vi "LV SciSDK INIT OSCILLOSCOPE.vi"(0 "Oscilloscope Name":string, 1 "Trigger Mode":string(combo)="self", 2 "Decimator":u32, 3 "Timeout":dbl=5000.0, 4 "Handle In":T2, 5 "error in (no error)":errorcluster, 6 "Pretrigger":u32, 7 "Acq Mode":string(combo)="blocking", 8 "Trigger Level":u32, 9 "Trigger Channel":u32, 10 "Trigger Polarity":string(combo)="pos", 11 "Auto Arm":u32=1) -> (18 "Oscilloscope Handle Out":T1, 19 "error out":errorcluster)   [LabVIEW 2021]
uses:
  SciSDK_Labview.lvlib
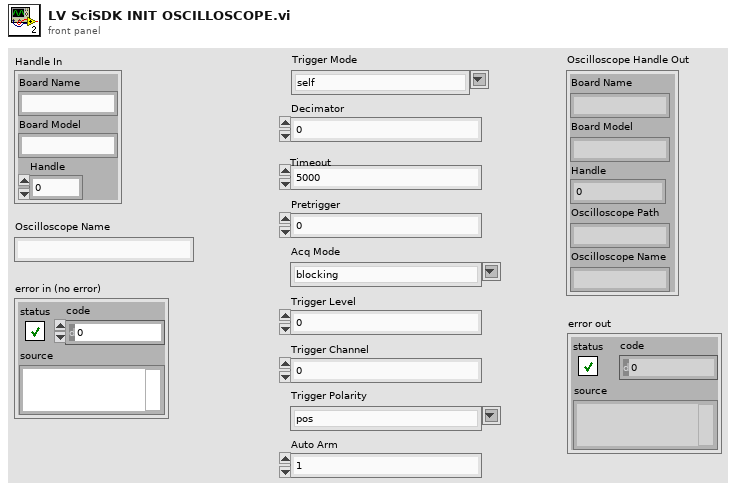
[diagram p1: front panel]
types:
  T1 = cluster{"Board Name":string, "Board Model":string, "Handle":u64, "Oscilloscope Path":string, "Oscilloscope Name":string}
  T2 = cluster{"Board Name":string, "Board Model":string, "Handle":u64}
  T3 = cluster{"Board Name":string, "Board Model":string, "Handle":u64, string, "Oscilloscope Name":string}
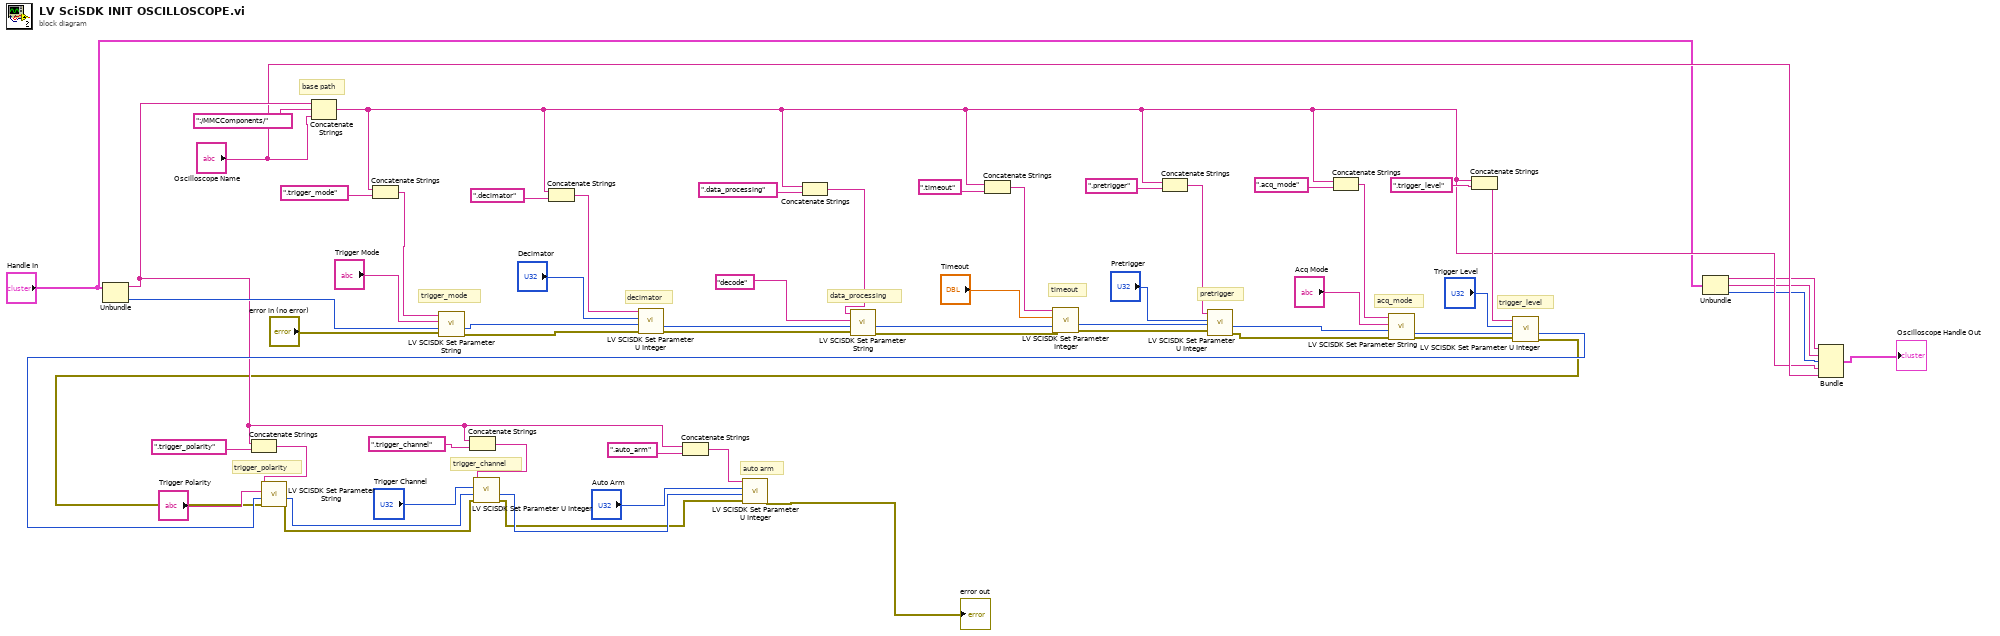
[diagram p0: block diagram]
diagram:
  # "auto arm"
  # "trigger_polarity"
  # "trigger_channel"
  # "trigger_level"
  # "acq_mode"
  # "pretrigger"
  # "base path"
  # "timeout"
  # "data_processing"
  # "decimator"
  # "trigger_mode"
  n1 = Unbundle("Handle In") -> ("Board Name"=w21:string, "Handle"=w60:u64)  [unwired: 1 out]
  n2 = Concatenate Strings(w21, ".trigger_polarity" ("string")) -> (w34:string)
  n3 = Concatenate Strings(w21, ":/MMCComponents/" ("string"), "Oscilloscope Name") -> (w17:string)
  n4 = Concatenate Strings(w17, ".trigger_mode" ("string")) -> (w54:string)
  n5 = call "LV SCISDK Set Parameter String.vi"("error in (no error)"="error in (no error)", "handle"=w60, "value"="Trigger Mode", "Path"=w54) -> ("error out"=w10:errorcluster, "handle out"=w59:u64)  [unwired: 5 in, 1 out]
  n6 = Concatenate Strings(w21, ".trigger_channel" ("string")) -> (w36:string)
  n7 = Concatenate Strings(w17, ".decimator" ("string")) -> (w52:string)
  n8 = call "LV SCISDK Set Parameter U Integer.vi"("error in (no error)"=w10, "handle"=w59, "value"="Decimator", "Path"=w52) -> ("error out"=w9:errorcluster, "handle out"=w58:u64)  [unwired: 5 in, 1 out]
  n9 = Concatenate Strings(w21, ".auto_arm" ("string")) -> (w20:string)
  n10 = Concatenate Strings(w17, ".data_processing" ("string")) -> (w47:string)
  n11 = call "LV SCISDK Set Parameter String.vi"("error in (no error)"=w9, "handle"=w58, "value"="decode", "Path"=w47) -> ("error out"=w8:errorcluster, "handle out"=w57:u64)  [unwired: 5 in, 1 out]
  n12 = Concatenate Strings(w17, ".timeout" ("string")) -> (w46:string)
  n13 = call "LV SCISDK Set Parameter Integer.vi"("error in (no error)"=w8, "handle"=w57, "value"="Timeout", "Path"=w46) -> ("error out"=w7:errorcluster, "handle out"=w45:u64)  [unwired: 5 in, 1 out]
  n14 = Concatenate Strings(w17, ".pretrigger" ("string")) -> (w44:string)
  n15 = call "LV SCISDK Set Parameter U Integer.vi"("error in (no error)"=w7, "handle"=w45, "value"="Pretrigger", "Path"=w44) -> ("error out"=w6:errorcluster, "handle out"=w39:u64)  [unwired: 5 in, 1 out]
  n16 = Concatenate Strings(w17, ".acq_mode" ("string")) -> (w40:string)
  n17 = call "LV SCISDK Set Parameter String.vi"("error in (no error)"=w6, "handle"=w39, "value"="Acq Mode", "Path"=w40) -> ("error out"=w5:errorcluster, "handle out"=w38:u64)  [unwired: 5 in, 1 out]
  n18 = Concatenate Strings(w17, ".trigger_level" ("string")) -> (w37:string)
  n19 = call "LV SCISDK Set Parameter U Integer.vi"("error in (no error)"=w5, "handle"=w38, "value"="Trigger Level", "Path"=w37) -> ("error out"=w4:errorcluster, "handle out"=w26:u64)  [unwired: 5 in, 1 out]
  n20 = call "LV SCISDK Set Parameter String.vi"("error in (no error)"=w4, "handle"=w26, "value"="Trigger Polarity", "Path"=w34) -> ("error out"=w3:errorcluster, "handle out"=w27:u64)  [unwired: 5 in, 1 out]
  n21 = call "LV SCISDK Set Parameter U Integer.vi"("error in (no error)"=w3, "handle"=w27, "value"="Trigger Channel", "Path"=w36) -> ("error out"=w2:errorcluster, "handle out"=w23:u64)  [unwired: 5 in, 1 out]
  n22 = call "LV SCISDK Set Parameter U Integer.vi"("error in (no error)"=w2, "handle"=w23, "value"="Auto Arm", "Path"=w20) -> ("error out"=→"error out":errorcluster)  [unwired: 5 in, 2 out]
  n23 = Unbundle("Handle In") -> ("Board Name"=w15:string, "Board Model"=w14:string, "Handle"=w13:u64)
  n24 = Bundle("Board Name"=w15, "Board Model"=w14, "Handle"=w13, w17, "Oscilloscope Name"="Oscilloscope Name") -> (→"Oscilloscope Handle Out":T3)  [unwired: 1 in]
